vi "HiResTime.vi"() -> ()   [LabVIEW 2016]
panel:
  out "relative seconds":dbl format="%_19f"
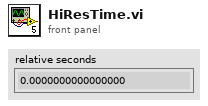
[diagram p1: front panel]
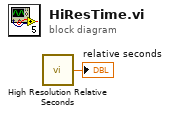
[diagram p0: block diagram]
diagram:
  n1 = call <vilib>:"High Resolution Relative Seconds.vi"() -> ("relative seconds"=→"relative seconds":dbl)
